vi "3.9.1-Diff.vi"(1 "Numeric":dbl) -> (0 "Numeric 2":dbl)   [LabVIEW 2010]
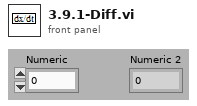
[diagram p1: front panel]
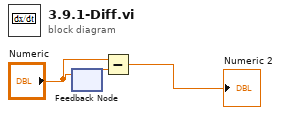
[diagram p0: block diagram]
diagram:
  n1 = feedback #1() -> (w1:dbl)  [unwired: 1 in]
  n2 = feedback-in #1("Numeric") -> ()
  n3 = Subtract(x="Numeric", y=w1) -> (x-y=→"Numeric 2":dbl)
